vi "Set Window Title.vi"(8 "error in (no error)":errorcluster, 10 "FP Window:Title":string, 11 "Station Actor in":refnum<class "Station Actor.lvclass">) -> (0 "error out":errorcluster, 3 "Station Actor out":refnum<class "Station Actor.lvclass">)   [LabVIEW 2019, in "Station Actor.lvlib" / "Station Actor.lvclass"]
uses:
  Station Actor.lvclass
  Station Actor.lvclass/Station Actor.ctl
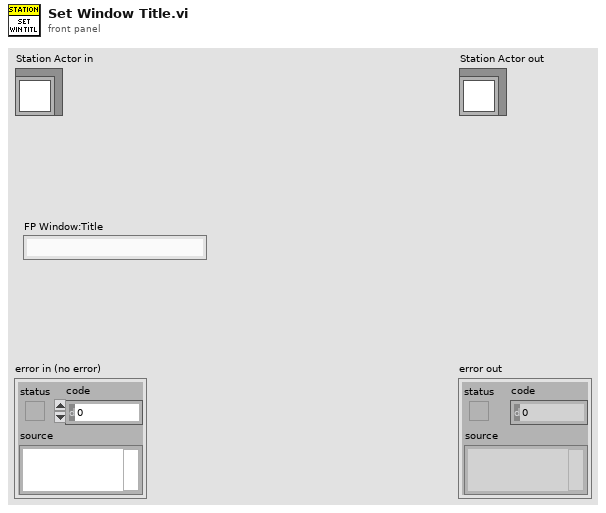
[diagram p1: front panel]
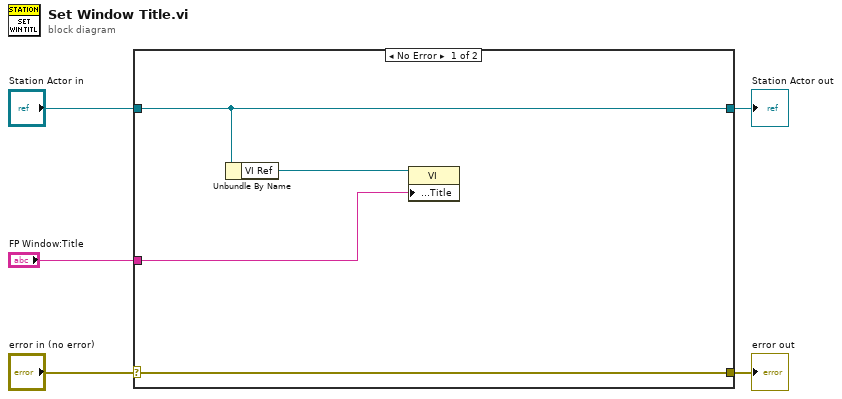
[diagram p0: block diagram]
diagram:
  n1 = case shown="No Error" "error in (no error)" {
    selector: "error in (no error)" -> [w9 w11]
    tunnel: [w9 w11] -> w4
    tunnel: [w8 w10] -> w2
    tunnel: "Station Actor in" -> [w8 w10]
    tunnel: "FP Window:Title" -> [w6 _]
    frame No Error {
      n2 = Unbundle By Name(w8) -> ("VI Ref"=w7:refnum<vi>)
      n3 = property class="VI"(reference=w7, "Front Panel.Title"=w6) -> ()  [unwired: 1 in, 2 out]
    }
    frame Error {
    }
  }
  "error out" <- w4
  "Station Actor out" <- w2
